vi "ESE.vi"(8 "error in (no error)":errorcluster, 10 "Node In":string, 11 "VISA resource name":refnum<visa-resource-name>) -> (0 "error out":errorcluster, 1 "ESE":dbl, 2 "Node Out":string, 3 "VISA resource name out":refnum<visa-resource-name>, 4 "Command String":string)   [LabVIEW 2013, in "Keithley 2600 Series.lvlib"]
doc: "Event Status Enable Register query. *ESE?\n\n<b>Functions and Attributes Used</b>\nstatus.standard.enable"
uses:
  Keithley 2600 Series.lvlib
panel:
  # "(c) 2008 Keithley Instruments, Inc.  ALL RIGHTS RESERVED."
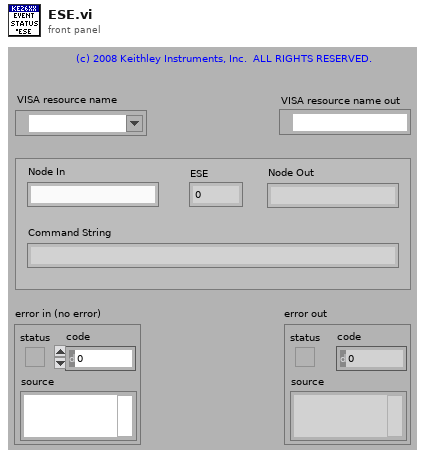
[diagram p1: front panel]
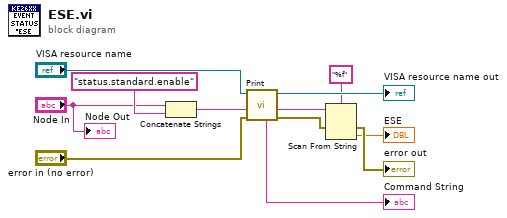
[diagram p0: block diagram]
diagram:
  n1 = Concatenate Strings("Node In", "status.standard.enable" ("string")) -> (w10:string)
  n2 = call "Print.vi"("error in (no error)"="error in (no error)", "Input"=w10, "VISA resource name"="VISA resource name") -> ("error out"=w4:errorcluster, "Output"=w6:string, "VISA resource name out"=→"VISA resource name out":refnum<visa-resource-name>, "Command String"=→"Command String":string)  [unwired: 2 in, 3 out]
  n3 = Scan From String(format string="%f", input string=w6, error in=w4) -> (error out=→"error out":errorcluster, output 1=→"ESE":dbl)  [unwired: 1 in, 3 out]
  "Node Out" <- "Node In"
